vi "DIOSerialTesting.vi"() -> ()   [LabVIEW 2016]
uses:
  FPGA/DIOSerialPort/DIOSerialPortSettings.ctl
  <vilib>/rvi/Emulation/niFpgaGetClockAttributes.vi
  <vilib>/rvi/Emulation/niFpgaSctlEmulationGetInTimedLoop.vi
  <vilib>/rvi/Emulation/niFpgaEmulationReportErrorSimple.vi
  <vilib>/rvi/Emulation/niFpgaEmulationIsFPGAContextNoSignature.vi
  <vilib>/rvi/errors/niFpgaSetErrorForExecOnDevCompSimple.vi
  <vilib>/rvi/eio/common/nirviEmuReportErrorAndStop.vi
  <vilib>/rvi/DataTransferAndStorage/Container/Common/niFpgaContainerGetUniqueNameForEmu.vi
  <vilib>/rvi/FIFO/Fifo_Resource/nirvififoEmulationSetSize.vi
  <vilib>/rvi/FIFO/Fifo_Resource/nirviFifoEmulationQueueMgr.vi
  <instcachedir>/0/nirviFifoEmulationQueueMgr_E5CAEC123FF24DC58D834DCA3CDAA9B5.lvgen/nirviFifoEmulationQueueMgr_E5CAEC123FF24DC58D834DCA3CDAA9B5_009.vi
  <vilib>/Utility/error.llb/Clear Errors.vi
  <vilib>/rvi/FIFO/Fifo_Resource/nirvififoEmulationCreateLock.vi
  <vilib>/rvi/Emulation/niFpgaProcessEmulError.vi
  <vilib>/rvi/FIFO/Fifo_Resource/nirvififoEmulationObtainLock.vi
  <vilib>/rvi/FIFO/Fifo_Resource/nirvififoEmulationReleaseLock.vi
  <vilib>/rvi/occurrence/nirviWaitOnOccurrenceBase.vi
  <vilib>/rvi/errors/nirviReportUnexpectedCaseInternalError.vi
  <vilib>/rvi/errors/nirviReportUnexpectedCaseInternalError (U32).vi
  <vilib>/rvi/Emulation/niFpgaCriticalErrorInLSC.vi
  <vilib>/rvi/FIFO/Fifo_Resource/nirvififoEmulationDetermineInputValidOut.vi
  <vilib>/rvi/DataTransferAndStorage/Container/XNode/niFpgaContainer.xnode
  <vilib>/rvi/FIFO/Fifo_Resource/nirvififoEmulationRead.vi
  <vilib>/rvi/FIFO/Fifo_Resource/nirvififoEmulationWrite.vi
panel:
  out "Bytes":i32
  out "Frames":i32
  out "Array":u8[](array[numeric]) format="%02x"
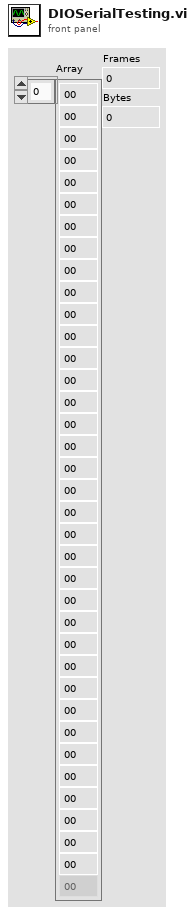
[diagram p1: front panel]
types:
  T1 = typedef "DIOSerialPortSettings.ctl" = cluster{"TxPort":refnum<k21>, "TxDataFIFO":refnum<k21>, "RxPort":refnum<k21>, "RxDataFIFO":refnum<k21>}
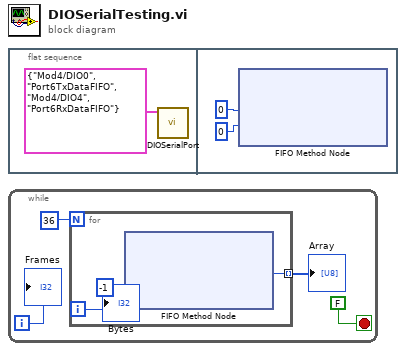
[diagram p0: block diagram]
diagram:
  n1 = flat-sequence {
    frame #0 {
      n2 = call "DIOSerialPort.vi"("DIOSerialPortSettings"=T1 {"TxPort"="Mod4/DIO0", "TxDataFIFO"="Port6TxDataFIFO", "RxPort"="Mod4/DIO4", "RxDataFIFO"="Port6RxDataFIFO"}) -> ()  [unwired: 11 in]
    }
    frame #1 {
      n3 = xnode ("FIFO Method Node")("Element"=u8 0, "Timeout"=0) -> ()  [unwired: 1 in, 2 out]
    }
  }
  n4 = while {
    i -> [w4]
    stop <- FALSE stop-if-true
    n5 = for {
      N: 36 -> [_]
      tunnel: [w9] -> w6 mode=indexing
      i -> [w8]
      n6 = xnode ("FIFO Method Node")("Timeout"=-1) -> ("Element"=w9:u8)  [unwired: 1 in, 2 out]
      "Bytes" <- w8
    }
    "Array" <- w6
    "Frames" <- w4
  }
